vi "Arrrduino close.vi"(1 "error in (no error)":errorcluster, 2 "VISA Refnum in":refnum<visa-resource-name>) -> ()   [LabVIEW 2014]
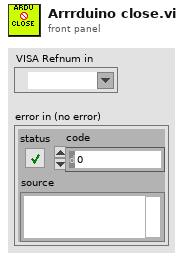
[diagram p1: front panel]
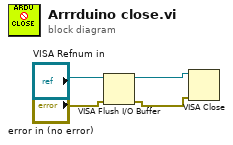
[diagram p0: block diagram]
diagram:
  n1 = VISA Flush I/O Buffer(VISA resource name="VISA Refnum in", error in (no error)="error in (no error)") -> (VISA resource name out=w4:refnum<visa-resource-name>, error out=w3:errorcluster)  [unwired: 1 in]
  n2 = VISA Close(VISA resource name=w4, error in (no error)=w3) -> ()  [unwired: 1 out]
